vi "RIMAS FITS Header Update Offsets.vi"(8 "Error In":errorcluster, 10 "Offsets":u16[](array[numeric]) format="%.0x", 11 "header file":string[](array[string])) -> (0 "Error Out":errorcluster, 3 "updated hdr file":string[](array[string]))   [LabVIEW 2021]
panel:
  out "String":string
  out "sample text":string="#----------------------------------------------------------------\n# Parameters\n#----------------------------------------------------------------\n# PAR      INIT               CMT\n  OBSMODE  TBD                photo, r30, r4000 observing mode\n  OBJNAME  TBD                name of object\n  OBJECT   TBD                name of object\n  OBSTYPE  TBD                object, flat, bias, etc.\n  IMAGETYP TBD                object, flat, bias, etc.\n  OBSERVER TBD                observer(s) \n  OBSAFFIL TBD                observer(s) affiliation\n  DATEOBS  TBD                UT date (yyyy-mm-dd) of observation\n  LST-OBS  TBD                Local Sidereal Time of exposure start\n  JD       0                  Julian day\n  UTCSTART TBD                universal time (start of exposure)\n  UT       TBD                universal time (start of exposure)\n  UTC      TBD                universal time (start of exposure)\n  UTCEND   TBD                universal time (end of exposure)\n  EXPTIMES 2000               exposure time in ms\n  EXPTIMEL 10000              exposure time in ms\n  WAVELENG TBD                (Fill in) \n  NFRAMES  2                  number of sample up-the ramp frames\n  NGROUPS  I       1                  number of sample groups\n  NDATA    I       0                  number of samples\n  FRAME_N  I       0                  current frame\n  DEVICE   S       TBD                Device of machine capturing this frame (0): YJ, (1): HK\n  TELRA    S       TBD                TCS right ascension (hh:mm:ss)\n  TELDEC   S       TBD                TCS declination (hh:mm:ss)\n  OBSRA    S       TBD                requested right ascension (hh:mm:ss)\n  OBSDEC   S       TBD                requested declination (hh:mm:ss)\n  RA       S       TBD                Right ascension (J2000)\n  DEC      S       TBD                Declination (J2000)\n  RAOFF    S       TBD                RA offset (J2000)\n  DECOFF   S       TBD                DEC offset (J2000)\n  ST       S       TBD                Local Sidereal Time\n  EQUINOX  F       2000               equinox of OBSRA and OBSDEC\n  AIRMASS  F       0                  airmass\n  FILTER0  S       TBD                Y, J, Open, None (corresponds to cam 0)\n  FILTER1  S       TBD                H, K, Open, None (corresponds to cam 1)\n  FILTER2  S       TBD                unknown (corresponds to specialty filter wheel, both cameras)\n  SLITWID  S       TBD                slit width in arcsec\n  FILTER   S       TBD                Composite Filter name\n  F0POS    S       TBD                Filter Position for FW0\n  F1POS    S       TBD                Filter Position for FW1\n  F2POS    S       TBD                Filter Position for FW2\n  S0POS    S       TBD                Slit Position for slit wheel\n  TRIMSEC  S       TBD                Valid pixels for extraction\n  CRVAL1   F       0                  RA for WCS Axis 1\n  CRVAL2   F       0                  DEC for WCS Axis 2\n  TELFOCUS S       TBD                telescope focus position\n  HA       S       TBD                hour angle\n  ZA       S       TBD                zenith angle\n  PARANGLE S       TBD                Parallactic Angle at start of exposure\n  INSTCVR  S       TBD                Status of instrument cover\n  TCSHLTH  S       TBD                Health of DCT TCS\n  ROTANGLE S       TBD                Cass. Rotator angle at exposure start\n  M1CVR    S       TBD                status of DCT M1 mirror cover\n  TCS_STAT S       TBD                State of DCT TCS\n  TELALT   S       TBD                Telescope Altitude at start of exposure\n  TELAZ    S       TBD                Telescope Azimuth at start of exposure\n  COMAZDIF S       TBD                Telescope-Dome Azimuth difference\n  DOMOCCUL S       TBD                Dome occultation warnming\n  GUIMODE  S       TBD                TCS guide mode\n  IPA      S       TBD                Instrument position angle (degrees)\n  PRESSURE S       TBD                Air pressure in mBars\n  TEMPAMB  S       TBD                Mean ambient temperature in deg C\n  TEMPDEW  S       TBD                Dew point in deg C\n  HUMIDITY S       TBD                Relative humidity, precent\n  WINDDIR  S       TBD                Mean wind direction in deg., N through E\n  WINDVEL  S       TBD                Mean wind speed in m/s\n  TEMP01   F       0                  temperature in K of X\n  TEMP02   F       0                  temperature in K of X\n  TEMP03   F       0                  temperature in K of X\n  TEMP04   F       0                  temperature in K of X\n  TEMP05   F       0                  temperature in K of X\n  TEMP06   F       0                  temperature in K of X\n  TEMP07   F       0                  temperature in K of X\n  TEMP08   F       0                  temperature in K of X\n  TEMP09   F       0                  temperature in K of X\n  TEMP10   F       0                  temperature in K of X\n  TEMP11   F       0                  temperature in K of X\n  TEMP12   F       0                  temperature in K of X\n  TEMP13   F       0                  temperature in K of X\n  TEMP14   F       0                  temperature in K of X\n  TEMP15   F       0                  temperature in K of X\n  TEMP16   F       0                  temperature in K of X\n  OFFV01   S       0x369              offset 01 val\n  OFFV02   S       0x361              offset 02 val\n  OFFV03   S       0x361              offset 03 val\n  OFFV04   S       0x363              offset 04 val\n  OFFV05   S       0x35a              offset 05 val\n  OFFV06   S       0x357              offset 06 val\n  OFFV07   S       0x360              offset 07 val\n  OFFV08   S       0x361              offset 08 val\n  OFFV09   S       0x34a              offset 09 val\n  OFFV10   S       0x34c              offset 10 val\n  OFFV11   S       0x347              offset 11 val\n  OFFV12   S       0x349              offset 12 val\n  OFFV13   S       0x34a              offset 13 val\n  OFFV14   S       0x34b              offset 14 val\n  OFFV15   S       0x349              offset 15 val\n  OFFV16   S       0x349              offset 16 val\n  OFFV17   S       0x351              offset 17 val\n  OFFV18   S       0x350              offset 18 val\n  OFFV19   S       0x353              offset 19 val\n  OFFV20   S       0x351              offset 20 val\n  OFFV21   S       0x351              offset 21 val\n  OFFV22   S       0x351              offset 22 val\n  OFFV23   S       0x350              offset 23 val\n  OFFV24   S       0x353              offset 24 val\n  OFFV25   S       0x350              offset 25 val\n  OFFV26   S       0x352              offset 26 val\n  OFFV27   S       0x353              offset 27 val\n  OFFV28   S       0x352              offset 28 val\n  OFFV29   S       0x353              offset 29 val\n  OFFV30   S       0x351              offset 30 val\n  OFFV31   S       0x351              offset 31 val\n  OFFV32   S       0x355              offset 32 val\n  FOCUS0   S       TBD                focus position of camera0\n  FOCUS1   S       TBD                focus position of camera1\n#----------------------------------------------------------------\n## Common Parameters\n##----------------------------------------------------------------\n# PAR      TYPE    INIT               CMT\n  TELESCOP S       DCT                Telescope name\n  INSTRUME S       RIMAS              instrument name\n  LATITUDE F       34.7443            latitude, degrees\n  LONGITUD F       -111.4223          east longitude, degrees\n  OBSREF   S       WGS84              The coordinate system for longitude and latitude\n  OBSALT   F       0                  altitude in meters\n  CD1_1    F       0                  WCS coordinate matrix\n  CD2_2    F       0                  WCS coordinate matrix\n  CD1_2    F       0                  WCS coordinate matrix\n  CD2_1    F       0                  WCS coordinate matrix\n  CTYPE1   S       RA---TAN           Axis type for WCS axis 1\n  CTYPE2   S       DEC--TAN           Axis type for WCS axis 2\n  CRPIX1   F       0                  Reference point along WCS Axis 1\n  CRPIX2   F       0                  Reference point along WCS Axis 2\n  CAMERA   S       TBD                0 (YJ) or 1 (HK)\n  GAIN     F       0                  (e-/ADU)\n  SATURATE F       0                  (ADU)\n  RDNOISE  F       0                  Read noise of camera\n  DETECTOR S       TBD                CMOS detector name\n  DETSIZE  S       2048x2048          detector size in pixels\n  BINNING  S       1x1                binning\n  BINX     S       1pixel             (Fill in)\n  BINY     S       1pixel             (Fill in)\n  PIXSCALE F       0                  pixel scale in arcsec/pixel for 1x1 binning\n"
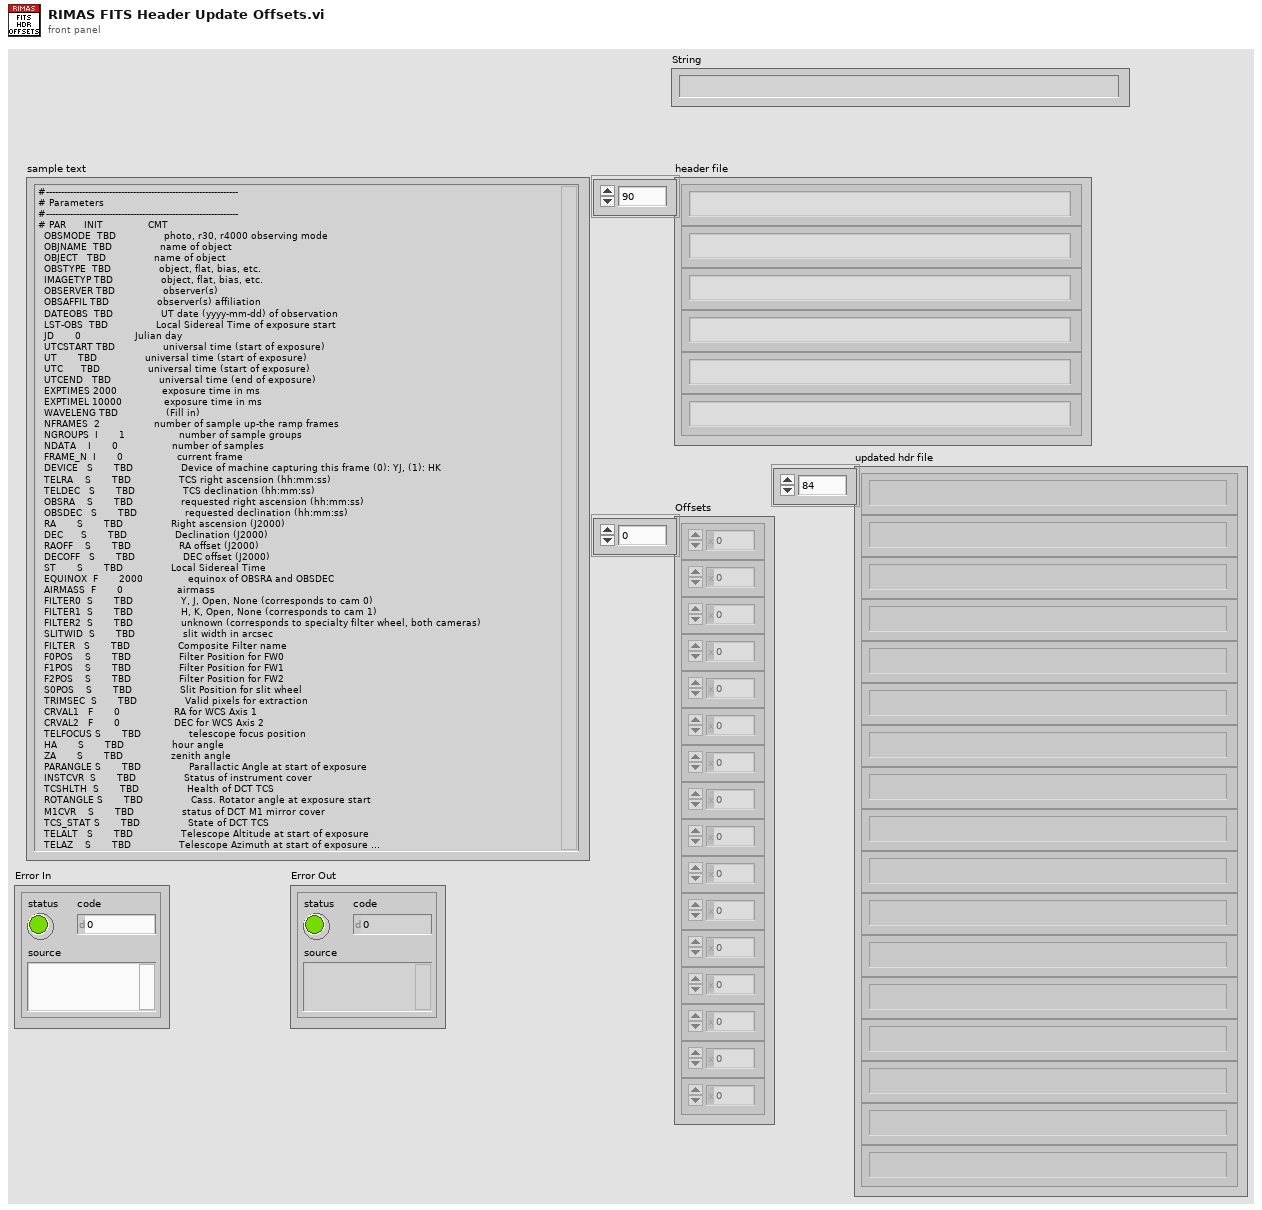
[diagram p1: front panel]
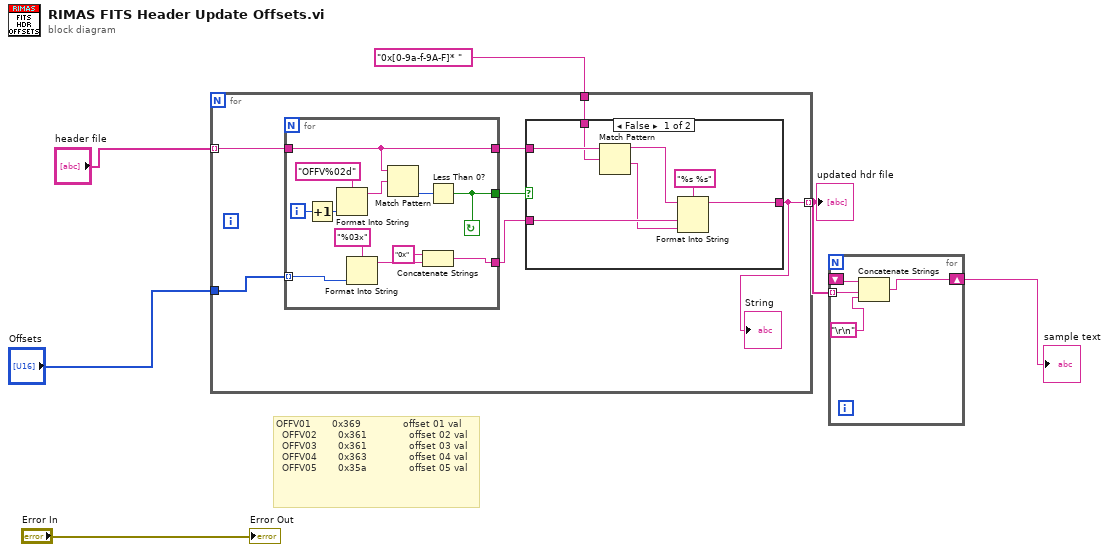
[diagram p0: block diagram]
diagram:
  # "OFFV01       0x369              offset 01 val\n  OFFV02       0x361              offset 02 val\n  OFFV03       0x361              offset 03 val\n  OFFV04       0x363              offset 04 val\n  OFFV05       0x35a              offset 05 val"
  n1 = for {
    tunnel: "Offsets" -> [w9]
    tunnel: "header file" -> [w13] mode=indexing
    tunnel: "0x[0-9a-f-9A-F]* " ("regular expression") -> [w10]
    tunnel: [w7] -> w2 mode=indexing
    n2 = for {
      tunnel: w13 -> [w32]
      tunnel: [w32] -> w11
      tunnel: [w31] -> w12
      tunnel: w9 -> [w29] mode=indexing
      tunnel: [w23] -> w8
      i -> [w26]
      stop <- w31 continue-if-true
      n3 = Increment(x=w26) -> (x+1=w28:i32)
      n4 = Format Into String(format string="OFFV%02d", w28) -> (resulting string=w25:string)  [unwired: 2 in, 1 out]
      n5 = Format Into String(format string="%03x", w29) -> (resulting string=w24:string)  [unwired: 2 in, 1 out]
      n6 = Match Pattern(string=w32, regular expression=w25) -> (offset past match=w33:i32)  [unwired: 1 in, 3 out]
      n7 = Concatenate Strings("0x" ("string"), w24) -> (w23:string)
      n8 = Less Than 0?(x=w33) -> (x < 0?=w31:bool)
    }
    n9 = case shown="False" w12 {
      tunnel: w11 -> [w20 w21]
      tunnel: w10 -> [w19 _]
      tunnel: w8 -> [w16 _]
      tunnel: [w14 w21] -> w7
      frame False {
        n10 = Match Pattern(string=w20, regular expression=w19) -> (before substring=w18:string, after substring=w15:string)  [unwired: 1 in, 2 out]
        n11 = Format Into String(format string="%s %s", initial string=w18, w16, w15) -> (resulting string=w14:string)  [unwired: 1 in, 1 out]
      }
      frame True {
      }
    }
    "String" <- w7
  }
  "updated hdr file" <- w2
  n12 = for {
    tunnel: w2 -> [w37] mode=indexing
    shift-right: [w35] -> w1
    shift-left: _ -> [w36]
    n13 = Concatenate Strings(w36, w37, "\r\n") -> (w35:string)
  }
  "sample text" <- w1
  "Error Out" <- "Error In"
